vi "Vision_Version_1.vi"(0 "Source Image":T2, 5 "Red or Hue":cluster{"Lower value":i32, "Upper value":i32}={"Lower value"=155, "Upper value"=245}, 7 "Green or saturation":cluster{"Lower value":i32, "Upper value":i32}={"Lower value"=148, "Upper value"=255}, 9 "Blue or luminance":cluster{"Lower value":i32, "Upper value":i32}={"Lower value"=9, "Upper value"=93}, 11 "Error in":errorcluster) -> (4 "Apply Convex Hull":T2(plugin-control), 8 "Image Data":T1, 15 "error out":errorcluster)   [LabVIEW 2017]
uses:
  <vilib>/vision/Image Controls.llb/IMAQ Image.ctl
  <vilib>/vision/NI_Vision_Development_Module.lvlib
panel:
  out "sum":dbl
  out "After RGB":T2(plugin-control)
  out "Original Image":T2(plugin-control)
  out "Noise Removed":T2(plugin-control)
  out "Number of Regions":i32
  out "Particle Measurements (Pixels)":dbl[][](array[numeric]) format="%.2f"
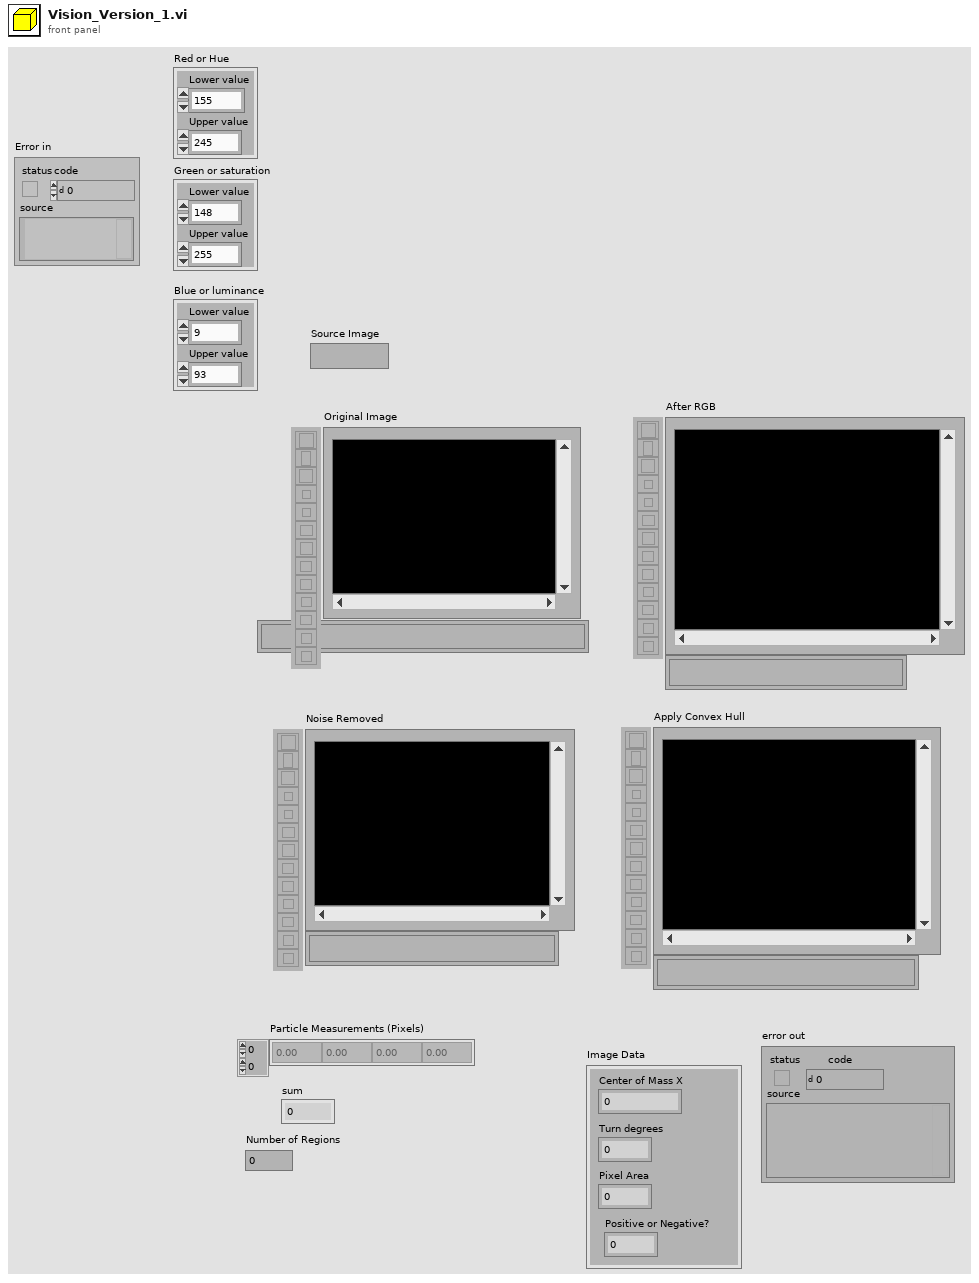
[diagram p1: front panel]
types:
  T1 = cluster{"Center of Mass X":dbl, "Turn degrees":dbl, "Pixel Area":dbl, "Positive or Negative?":dbl}
  T2 = typedef "IMAQ Image.ctl" = refnum<image>
  T3 = typedef "Particle Parameters" = i32
  T4 = cluster{"Measurement Parameter":T3, dbl, dbl, bool, bool}
  T5 = cluster{"Measurement Parameter":T3, dbl, dbl, bool, bool}[]
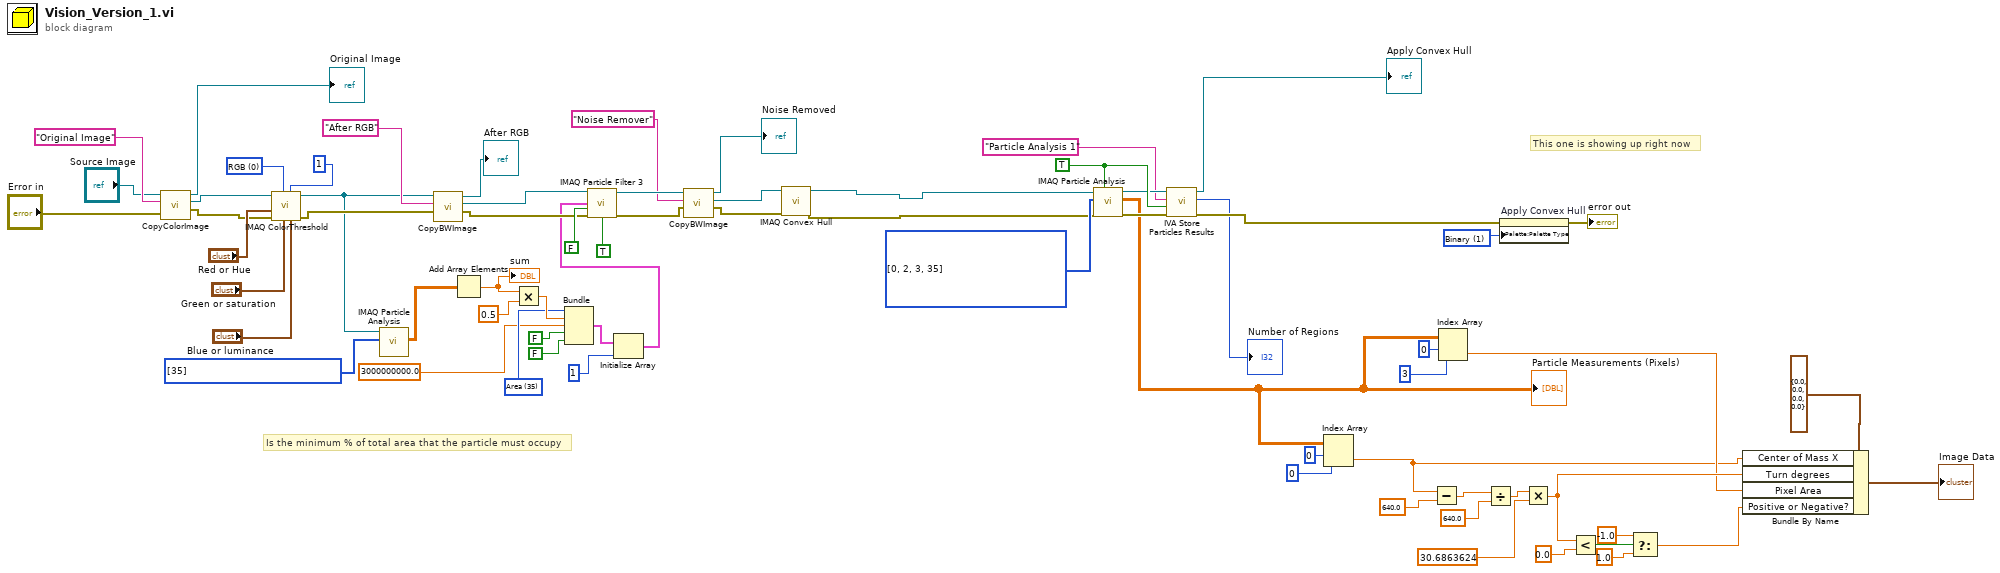
[diagram p0: block diagram]
diagram:
  w27 = T3 35 items=["Center of Mass X", "Center of Mass Y", "First Pixel X", "First Pixel Y", "Bounding Rect Left", "Bounding Rect Top", "Bounding Rect Right", "Bounding Rect Bottom", "Max Feret Diameter Start X", "Max Feret Diameter Start Y", "Max Feret Diameter End X", "Max Feret Diameter End Y", "Max Horiz. Segment Length Left", "Max Horiz. Segment Length Right", "Max Horiz. Segment Length Row", "-", "Bounding Rect Width", "Bounding Rect Height", "Bounding Rect Diagonal", "Perimeter", "Convex Hull Perimeter", "Holes' Perimeter", "Max Feret Diameter", "Equivalent Ellipse Major Axis", "Equivalent Ellipse Minor Axis", "Equivalent Ellipse Minor Axis (Feret)", "Equivalent Rect Long Side", "Equivalent Rect Short Side", "Equivalent Rect Diagonal", "Equivalent Rect Short Side (Feret)", "Average Horiz. Segment Length", "Average Vert. Segment Length", "Hydraulic Radius", "Waddel Disk Diameter", "-", "Area", "Holes' Area", "Particle & Holes' Area", "Convex Hull Area", "Image Area", "-", "Number of Holes", "Number of Horiz. Segments", "Number of Vert. Segments", "-", "Orientation", "Max Feret Diameter Orientation", "-", "% Area/Image Area", "% Area/(Particle & Holes' Area)", "Ratio of Equivalent Ellipse Axes", "Ratio of Equivalent Rect Sides", "-", "Elongation Factor", "Compactness Factor", "Heywood Circularity Factor", "Type Factor", "-", "Sum X", "Sum Y", "Sum XX", "Sum XY", "Sum YY", "Sum XXX", "Sum XXY", "Sum XYY", "Sum YYY", "-", "Moment of Inertia XX", "Moment of Inertia XY", "Moment of Inertia YY", "Moment of Inertia XXX", "Moment of Inertia XXY", "Moment of Inertia XYY", "Moment of Inertia YYY", "Norm. Moment of Inertia XX", "Norm. Moment of Inertia XY", "Norm. Moment of Inertia YY", "Norm. Moment of Inertia XXX", "Norm. Moment of Inertia XXY", "Norm. Moment of Inertia XYY", "Norm. Moment of Inertia YYY", "Hu Moment 1", "Hu Moment 2", "Hu Moment 3", "Hu Moment 4", "Hu Moment 5", "Hu Moment 6", "Hu Moment 7"] ("Measurement Parameter")
  w34 = i32[] [35] items=["Center of Mass X", "Center of Mass Y", "First Pixel X", "First Pixel Y", "Bounding Rect Left", "Bounding Rect Top", "Bounding Rect Right", "Bounding Rect Bottom", "Max Feret Diameter Start X", "Max Feret Diameter Start Y", "Max Feret Diameter End X", "Max Feret Diameter End Y", "Max Horiz. Segment Length Left", "Max Horiz. Segment Length Right", "Max Horiz. Segment Length Row", "-", "Bounding Rect Width", "Bounding Rect Height", "Bounding Rect Diagonal", "Perimeter", "Convex Hull Perimeter", "Holes' Perimeter", "Max Feret Diameter", "Equivalent Ellipse Major Axis", "Equivalent Ellipse Minor Axis", "Equivalent Ellipse Minor Axis (Feret)", "Equivalent Rect Long Side", "Equivalent Rect Short Side", "Equivalent Rect Diagonal", "Equivalent Rect Short Side (Feret)", "Average Horiz. Segment Length", "Average Vert. Segment Length", "Hydraulic Radius", "Waddel Disk Diameter", "-", "Area", "Holes' Area", "Particle & Holes' Area", "Convex Hull Area", "Image Area", "-", "Number of Holes", "Number of Horiz. Segments", "Number of Vert. Segments", "-", "Orientation", "Max Feret Diameter Orientation", "-", "% Area/Image Area", "% Area/(Particle & Holes' Area)", "Ratio of Equivalent Ellipse Axes", "Ratio of Equivalent Rect Sides", "-", "Elongation Factor", "Compactness Factor", "Heywood Circularity Factor", "Type Factor", "-", "Sum X", "Sum Y", "Sum XX", "Sum XY", "Sum YY", "Sum XXX", "Sum XXY", "Sum XYY", "Sum YYY", "-", "Moment of Inertia XX", "Moment of Inertia XY", "Moment of Inertia YY", "Moment of Inertia XXX", "Moment of Inertia XXY", "Moment of Inertia XYY", "Moment of Inertia YYY", "Norm. Moment of Inertia XX", "Norm. Moment of Inertia XY", "Norm. Moment of Inertia YY", "Norm. Moment of Inertia XXX", "Norm. Moment of Inertia XXY", "Norm. Moment of Inertia XYY", "Norm. Moment of Inertia YYY", "Hu Moment 1", "Hu Moment 2", "Hu Moment 3", "Hu Moment 4", "Hu Moment 5", "Hu Moment 6", "Hu Moment 7"] ("Pixel Measurements")
  w36 = u16 0 items=["RGB", "HSL", "HSV", "HSI"] ("Color Mode")
  w61 = u32 1 items=["Grayscale", "Binary", "Gradient", "Rainbow", "Temperature", "User Defined", "Binary 16 Bit", "Gradient 16 Bit", "Rainbow 16 Bit", "Temperature 16 Bit", "User Defined 16 Bit"] ("Palette Type")
  w68 = i32[] [0, 2, 3, 35] items=["Center of Mass X", "Center of Mass Y", "First Pixel X", "First Pixel Y", "Bounding Rect Left", "Bounding Rect Top", "Bounding Rect Right", "Bounding Rect Bottom", "Max Feret Diameter Start X", "Max Feret Diameter Start Y", "Max Feret Diameter End X", "Max Feret Diameter End Y", "Max Horiz. Segment Length Left", "Max Horiz. Segment Length Right", "Max Horiz. Segment Length Row", "-", "Bounding Rect Width", "Bounding Rect Height", "Bounding Rect Diagonal", "Perimeter", "Convex Hull Perimeter", "Holes' Perimeter", "Max Feret Diameter", "Equivalent Ellipse Major Axis", "Equivalent Ellipse Minor Axis", "Equivalent Ellipse Minor Axis (Feret)", "Equivalent Rect Long Side", "Equivalent Rect Short Side", "Equivalent Rect Diagonal", "Equivalent Rect Short Side (Feret)", "Average Horiz. Segment Length", "Average Vert. Segment Length", "Hydraulic Radius", "Waddel Disk Diameter", "-", "Area", "Holes' Area", "Particle & Holes' Area", "Convex Hull Area", "Image Area", "-", "Number of Holes", "Number of Horiz. Segments", "Number of Vert. Segments", "-", "Orientation", "Max Feret Diameter Orientation", "-", "% Area/Image Area", "% Area/(Particle & Holes' Area)", "Ratio of Equivalent Ellipse Axes", "Ratio of Equivalent Rect Sides", "-", "Elongation Factor", "Compactness Factor", "Heywood Circularity Factor", "Type Factor", "-", "Sum X", "Sum Y", "Sum XX", "Sum XY", "Sum YY", "Sum XXX", "Sum XXY", "Sum XYY", "Sum YYY", "-", "Moment of Inertia XX", "Moment of Inertia XY", "Moment of Inertia YY", "Moment of Inertia XXX", "Moment of Inertia XXY", "Moment of Inertia XYY", "Moment of Inertia YYY", "Norm. Moment of Inertia XX", "Norm. Moment of Inertia XY", "Norm. Moment of Inertia YY", "Norm. Moment of Inertia XXX", "Norm. Moment of Inertia XXY", "Norm. Moment of Inertia XYY", "Norm. Moment of Inertia YYY", "Hu Moment 1", "Hu Moment 2", "Hu Moment 3", "Hu Moment 4", "Hu Moment 5", "Hu Moment 6", "Hu Moment 7"] ("Pixel Measurements")
  w67 = TRUE ("Connectivity 4/8 (8)")
  # "Is the minimum % of total area that the particle must occupy"
  # "This one is showing up right now"
  n1 = call "CopyColorImage.vi"("Error in 1"="Error in", "Image Name"="Original Image", "Image"="Source Image") -> ("error out 2"=w38:errorcluster, "Out 2"=w51:T2, "Out"=→"Original Image":T2)  [unwired: 5 in, 1 out]
  n2 = call "IMAQ ColorThreshold"("Blue or Luma or Val or Inten Range"="Blue or luminance", "Replace Value"=1, "Green or Sat Range"="Green or saturation", "Color Mode"=w36, "error in (no error)"=w38, "Red or Hue Range"="Red or Hue", "Image Src"=w51) -> ("error out"=w46:errorcluster, "Image Dst Out"=w35:T2)  [unwired: 1 in, 2 out]
  n3 = call "IMAQ Particle Analysis"("Pixel Measurements"=w34, "Image"=w35) -> ("Particle Measurements (Pixels)"=w33:dbl[][])  [unwired: 3 in, 6 out]
  n4 = call "CopyBWImage.vi"("Error in 1"=w46, "Image Name"="After RGB", "Image"=w35) -> ("error out 2"=w49:errorcluster, "Out 2"=w50:T2, "Out"=→"After RGB":T2)  [unwired: 5 in, 1 out]
  n5 = Add Array Elements(numeric array=w33) -> (sum=w32:dbl)
  "sum" <- w32
  n6 = Multiply(x=w32, y=0.5) -> (x*y=w30:dbl)
  n7 = Bundle("Measurement Parameter"=w27, w30, 3000000000.0, FALSE, FALSE) -> (w29:T4)  [unwired: 1 in]
  n8 = Initialize Array(w29, 1 ("dimension size")) -> (w23:T5)
  n9 = call "IMAQ Particle Filter 3"("Image Src"=w50, "Selection Values"=w23, "Keep/Remove Particles (F)"=FALSE, "error in (no error)"=w49, "Fill Holes? (F)"=TRUE) -> ("Image Dst Out"=w43:T2, "error out"=w42:errorcluster)  [unwired: 8 in, 1 out]
  n10 = call "CopyBWImage.vi"("Error in 1"=w42, "Image Name"="Noise Remover", "Image"=w43) -> ("error out 2"=w44:errorcluster, "Out 2"=w45:T2, "Out"=→"Noise Removed":T2)  [unwired: 5 in, 1 out]
  n11 = call "IMAQ Convex Hull"("error in (no error)"=w44, "Image Src"=w45) -> ("error out"=w53:errorcluster, "Image Dst Out"=w54:T2)  [unwired: 8 in]
  n12 = call "IMAQ Particle Analysis"("Connectivity 4/8 (8)"=w67, "error in (no error)"=w53, "Pixel Measurements"=w68, "Image"=w54) -> ("error out"=w64:errorcluster, "Particle Measurements (Pixels)"=w11:dbl[][], "Image Out (duplicate)"=w66:T2)  [unwired: 1 in, 4 out]
  "Particle Measurements (Pixels)" <- w11
  n13 = call <vilib>:"IVA Store Particles Results.vi"("error in (no error)"=w64, "Connectivity 4/8 (8)"=w67, "Step Name"="Particle Analysis 1", "Image in"=w66) -> ("error out"=w63:errorcluster, "Number of Particles"=→"Number of Regions":i32, "Image dup"=→"Apply Convex Hull":T2)  [unwired: 5 out]
  n14 = Index Array(array=w11, index (row)=0, index (col)=0 ("disabled index (col)")) -> (element=w1:dbl)
  n15 = Subtract(x=w1, y=640.0) -> (x-y=w19:dbl)
  n16 = Index Array(array=w11, index (row)=0, index (col)=3 ("disabled index (col)")) -> (element=w2:dbl)
  n17 = Divide(x=w19, y=640.0) -> (x/y=w17:dbl)
  n18 = property on="Apply Convex Hull" class="ImageControl"(error in=w63, "Palette:Palette Type"=w61) -> (error out=→"error out":errorcluster)  [unwired: 1 in, 1 out]
  n19 = Multiply(x=w17, y=30.6863624) -> (x*y=w3:dbl)
  n20 = Less?(x=w3, y=0.0) -> (x < y?=w15:bool)
  n21 = Select(t=-1.0, s=w15, f=1.0) -> (s? t:f=w4:dbl)
  n22 = Bundle By Name(cluster=T1 {"Center of Mass X"=0.0, "Turn degrees"=0.0, "Pixel Area"=0.0, "Positive or Negative?"=0.0} ("Cluster"), "Center of Mass X"=w1, "Turn degrees"=w3, "Pixel Area"=w2, "Positive or Negative?"=w4) -> (→"Image Data":T1)
